vi "1 (SubVI).vi"(10 "Scalar":dbl, 11 "Numeric":dbl) -> (3 "Cluster":cluster{dbl[], dbl[]})   [LabVIEW 2020]
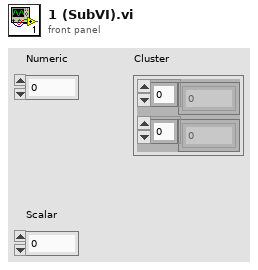
[diagram p1: front panel]
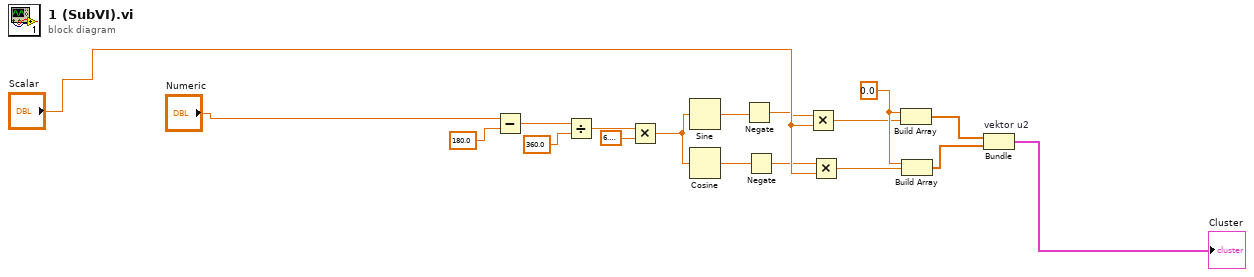
[diagram p0: block diagram]
diagram:
  w15 = 0.0 ("element")
  n1 = Subtract(x="Numeric", y=180.0) -> (x-y=w3:dbl)
  n2 = Divide(x=w3, y=360.0) -> (x/y=w5:dbl)
  n3 = Multiply(x=w5, y=6.283185307179586) -> (x*y=w7:dbl)
  n4 = Sine(x=w7) -> (sin(x)=w8:dbl)
  n5 = Cosine(x=w7) -> (cos(x)=w9:dbl)
  n6 = Negate(x=w8) -> (-x=w11:dbl)
  n7 = Negate(x=w9) -> (-x=w10:dbl)
  n8 = Multiply(x=w11, y="Scalar") -> (x*y=w14:dbl)
  n9 = Multiply(x=w10, y="Scalar") -> (x*y=w13:dbl)
  n10 = Build Array(w15, w14) -> (w16:dbl[])
  n11 = Build Array(w15, w13) -> (w17:dbl[])
  n12 = Bundle "vektor u2"(w16, w17) -> (→"Cluster":cluster{dbl[], dbl[]})  [unwired: 1 in]
